vi "Current Elevator State.vi"(8 "error in (no error)":errorcluster, 10 "Elevator State":T1 {"Current Elevation" scale=0.0..100.0; "Current Travel Rate" scale=-1.0..1.0}, 11 "EL-Go To Height in":refnum<class "EL-Go To Height.lvclass">) -> (0 "error out":errorcluster, 3 "EL-Go To Height out":refnum<class "EL-Go To Height.lvclass">)   [LabVIEW 2014, in "Elevator.lvlib" / "EL-Go To Height.lvlib" / "EL-Go To Height.lvclass"]
uses:
  EL-Go To Height.lvclass
  Elevator Class/Elevator State.ctl
  Elevator Class/Elevator.lvclass
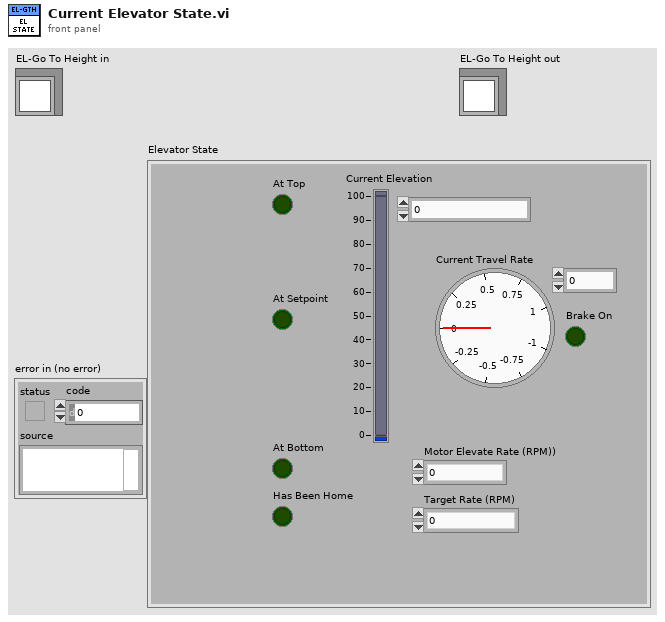
[diagram p1: front panel]
types:
  T1 = typedef "Elevator.lvlib/Elevator.lvclass/Elevator State.ctl" = cluster{"At Bottom":bool, "At Top":bool, "At Setpoint":bool, "Target Rate (RPM)":dbl, "Current Travel Rate":dbl, "Current Elevation":dbl, "Brake On":bool, "Motor Elevate Rate (RPM))":dbl, "Has Been Home":bool}
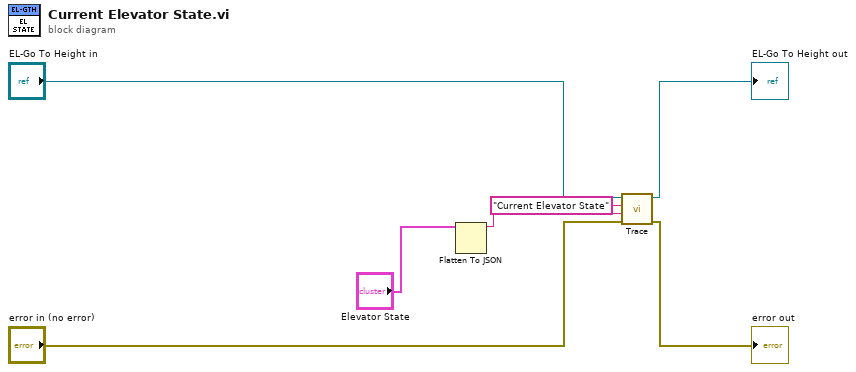
[diagram p0: block diagram]
diagram:
  n1 = Flatten To JSON(anything="Elevator State") -> (JSON string=w2:string)  [unwired: 2 in, 1 out]
  n2 = call-dynamic "Trace.vi"("error in (no error)"="error in (no error)", "Command Message"=w2, "Command Action"="Current Elevator State", "Command Actor in"="EL-Go To Height in") -> ("error out"=→"error out":errorcluster, "Command Actor out"=→"EL-Go To Height out":refnum<class "EL-Go To Height.lvclass">)  [unwired: 6 in]
